vi "Begin.vi"() -> (0 "error out":errorcluster, 1 "error out 2":errorcluster)   [LabVIEW 2013]
doc: "Called before other user functions, this VI is expected to open initial I/O refnums, load in file data, and do all program initialization. Notice that the <B>error out</B> terminal is simply used for data flow. Wiring it to other structures or subVIs ensures that this VI runs first."
uses:
  <vilib>/Rock Robotics/WPI/DriverStation/WPI_DriverStationRobotMode2.ctl
  <vilib>/Rock Robotics/SystemInterfaces/DIO/FPGA_DIOPWMChannel.ctl
  <vilib>/Rock Robotics/WPI/SafetyOutput/WPI_SafetyOutputConfigMenu.ctl
  <vilib>/Rock Robotics/WPI/Joystick/WPI_JoystickDeviceEnum.ctl
  <vilib>/Rock Robotics/SystemInterfaces/Typedef/FPGA_TypedefDigitalModule.ctl
  <vilib>/Rock Robotics/WPI/Solenoid/WPI_SolenoidChannel.ctl
  <vilib>/Rock Robotics/SystemInterfaces/DIO/FPGA_DIORelayChannel.ctl
  <vilib>/Rock Robotics/SystemInterfaces/DIO/FPGA_DIOChannel.ctl
  <vilib>/Rock Robotics/SystemInterfaces/AI/FPGA_AIChannel.ctl
  <vilib>/Rock Robotics/SystemInterfaces/Typedef/FPGA_TypedefAnalogModule.ctl
  <vilib>/Rock Robotics/WPI/Relay/WPI_RelayValue.ctl
  <vilib>/Rock Robotics/WPI/Relay/WPI_RelayDirection.ctl
  <vilib>/Rock Robotics/SystemInterfaces/Typedef/FPGA_TypedefSolenoidModule.ctl
  <vilib>/Rock Robotics/WPI/Solenoid/WPI_SolenoidValue.ctl
  Robot Global Data.vi
  <vilib>/Rock Robotics/WPI/RobotDrive/WPI_RobotDriveOpen2MotorWithTalon.vi
  <vilib>/Rock Robotics/WPI/MotorControl/WPI_MotorControlOpen Jaguar.vi
  <vilib>/Rock Robotics/WPI/Solenoid/WPI_SolenoidOpenDouble.vi
  <vilib>/Rock Robotics/WPI/MotorControl/WPI_MotorControlOpen Talon.vi
  <vilib>/Rock Robotics/WPI/Solenoid/WPI_SolenoidOpenSingle.vi
  <vilib>/Rock Robotics/WPI/Solenoid/WPI_SolenoidGetEnum.vi
  <vilib>/Rock Robotics/WPI/Solenoid/WPI_SolenoidSetEnum.vi
  <vilib>/Rock Robotics/WPI/Compressor/WPI_CompressorGetSetRefNum.vi
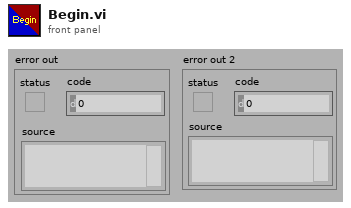
[diagram p1: front panel]
types:
  T1 = typedef "WPI_SolenoidValue.ctl" = enum16{"Off", "On", "Forward", "Reverse"}
  T2 = typedef "WPI_SolenoidChannel.ctl" = enum8{"Solenoid 1", "Solenoid 2", "Solenoid 3", "Solenoid 4", "Solenoid 5", "Solenoid 6", "Solenoid 7", "Solenoid 8", "Invalid"}
  T3 = typedef "FPGA_TypedefSolenoidModule.ctl" = enum16{"Solenoid Module 1", "Solenoid Module 2"}
  T4 = typedef "WPI_RelayDirection.ctl" = enum16{"Both directions", "Forward only", "Reverse only"}
  T5 = typedef "FPGA_DIORelayChannel.ctl" = enum8{"Relay 1", "Relay 2", "Relay 3", "Relay 4", "Relay 5", "Relay 6", "Relay 7", "Relay 8", "Invalid"}
  T6 = typedef "FPGA_TypedefDigitalModule.ctl" = enum16{"Digital Module 1", "Digital Module 2"}
  T7 = typedef "WPI_RelayValue.ctl" = enum16{"Off", "On", "Forward", "Reverse"}
  T8 = typedef "FPGA_DIOChannel.ctl" = enum8{"DIO 1", "DIO 2", "DIO 3", "DIO 4", "DIO 5", "DIO 6", "DIO 7", "DIO 8", "DIO 9", "DIO 10", "DIO 11", "DIO 12", "DIO 13", "DIO 14", "Invalid"}
  T9 = typedef "FPGA_AIChannel.ctl" = enum8{"AI 1", "AI 2", "AI 3", "AI 4", "AI 5", "AI 6", "AI 7", "AI 8", "Invalid"}
  T10 = typedef "FPGA_TypedefAnalogModule.ctl" = enum16{"Analog Module 1", "Analog Module 2"}
  T11 = typedef "FPGA_DIOPWMChannel.ctl" = enum8{"PWM 1", "PWM 2", "PWM 3", "PWM 4", "PWM 5", "PWM 6", "PWM 7", "PWM 8", "PWM 9", "PWM 10", "Invalid"}
  T12 = typedef "WPI_JoystickDeviceEnum.ctl" = enum16{"USB 1", "USB 2", "USB 3", "USB 4", "Kinect 1", "Kinect 2"}
  T13 = typedef "WPI_SafetyOutputConfigMenu.ctl" = enum16{"Enable", "Disable"}
  T14 = typedef "WPI_DriverStationRobotMode2.ctl" = enum16{"Autonomous Disabled", "Autonomous Enabled", "Teleop Disabled", "Teleop Enabled", "Timeout", "Finish", "Test Disabled", "Test Enabled"}
  T15 = typedef "WPI_MotorControlDeviceRef.ctl" = cluster{"DeviceStatus":errorcluster, "Type":enum16{"PWM", "CAN"}, "PWM":cluster{"Digital Module":T6, "PWM Channel":T11, "DeadBand":T16}, "CAN":cluster{"Device Number":u8, "Control Mode":T17, "Semaphore":T18, "Max Vout":dbl}, "Invert":bool, "TransformRef":T19, "InvTransformRef":T19}
  T16 = typedef "WPI_PWMDeadband.ctl" = cluster{"Name":string, "maxPositivePwm":i32, "minPositivePwm":i32, "centerPwm":i32, "maxNegativePwm":i32, "minNegativePwm":i32, "angularRange":u16}
  T17 = typedef "WPI_CANJaguar_ControlMode.ctl" = enum8{"Percent VBus", "Current", "Speed", "Position", "Voltage"}
  T18 = typedef "Semaphore RefNum" = refnum<k1>
  T19 = typedef "WPI_PWMTransform_ConPane.ctl" = refnum<vi>
  T20 = typedef "WPI_JoystickDevRef.ctl" = cluster{"Device":T12}
  T21 = typedef "WPI_DigitalInputDevRef.ctl" = cluster{"DevStatus":errorcluster, "DIO Channel":T8, "Digital Module":T6}
  T22 = typedef "WPI_RobotDriveDevRef.ctl" = cluster{"DevStatus":errorcluster, "Motors[]":T15[], "Square Inputs":bool, "Max Output":dbl, "Isochronous":bool}
  T23 = typedef "WPI_SolenoidDevRef.ctl" = cluster{"DevStatus":errorcluster, "Solenoid Module":T3, "Forward Solenoid Channel":T2, "Reverse Solenoid Channel":T2}
  T24 = typedef "WPI_RelayDevRef.ctl" = cluster{"DevStatus":errorcluster, "Relay Channel":T5, "Digital Module":T6, "Relay Direction":T4}
  T25 = typedef "WPI_CompressorDevRef.ctl" = cluster{"DevStatus":errorcluster, "DigitalInputDevRef":T21, "RelayDevRef":T24}
  T26 = typedef "WPI_AnalogChannelDevRef.ctl" = cluster{"DevStatus":errorcluster, "Analog Module":T10, "Analog Channel":T9}
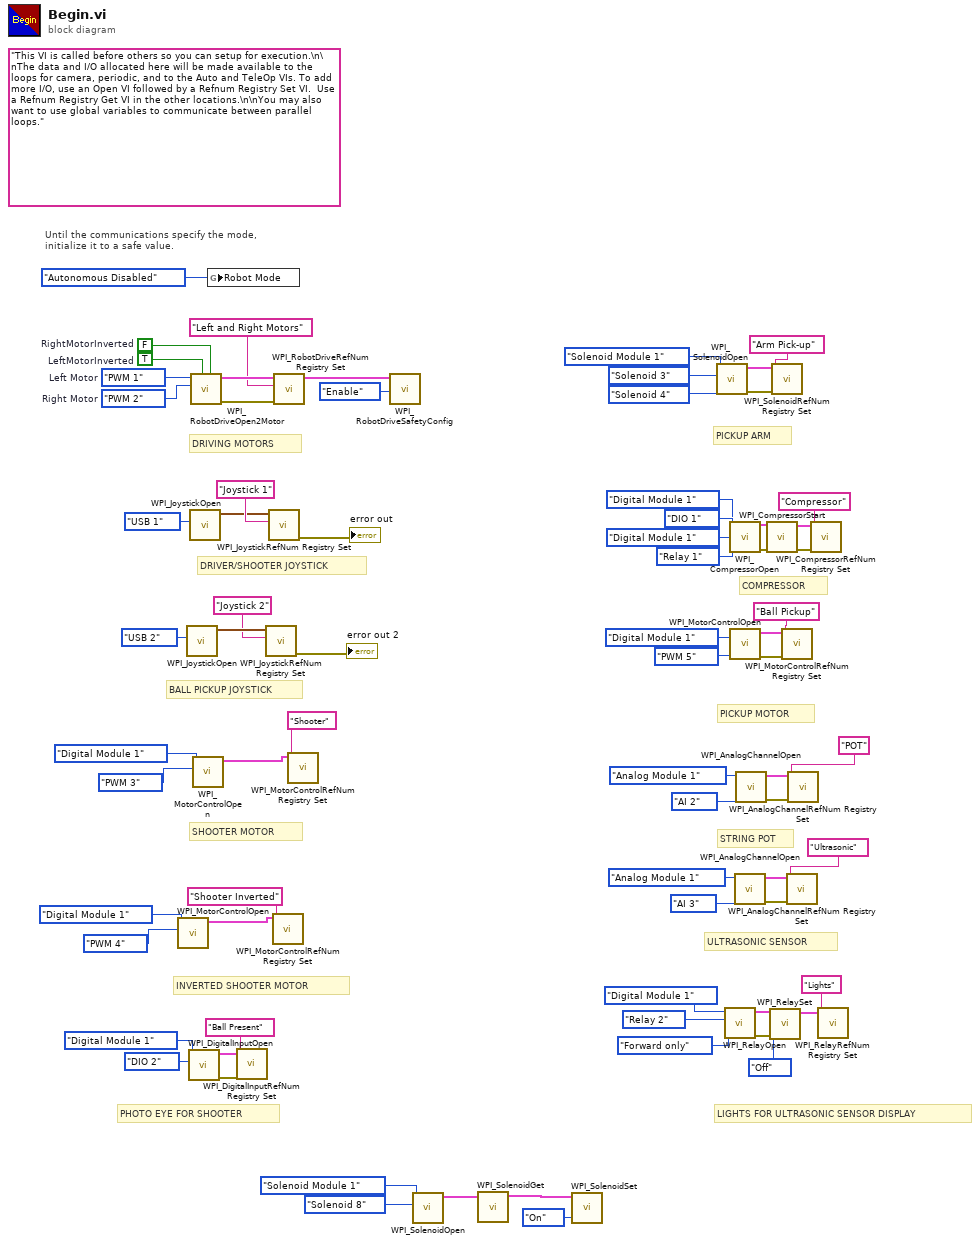
[diagram p0: block diagram]
diagram:
  w67 = FPGA_DIOPWMChannel."PWM 2"  # Right Motor
  w68 = FPGA_DIOPWMChannel."PWM 1"  # Left Motor
  w72 = TRUE  # LeftMotorInverted
  w73 = FALSE  # RightMotorInverted
  (unwired) "This VI is called before others so you can setup for execution.\n\nThe data and I/O allocated here will be made available to the loops for camera, periodic, and to the Auto and TeleOp VIs. To add more I/O, use an Open VI followed by a Refnum Registry Set VI.  Use a Refnum Registry Get VI in the other locations.\n\nYou may also want to use global variables to communicate between parallel loops."
  # "LIGHTS FOR ULTRASONIC SENSOR DISPLAY"
  # "PHOTO EYE FOR SHOOTER"
  # "ULTRASONIC SENSOR"
  # "STRING POT"
  # "PICKUP MOTOR"
  # "COMPRESSOR"
  # "PICKUP ARM"
  # "INVERTED SHOOTER MOTOR"
  # "SHOOTER MOTOR"
  # "BALL PICKUP JOYSTICK"
  # "DRIVER/SHOOTER JOYSTICK"
  # "DRIVING MOTORS"
  # "Until the communications specify the mode,\ninitialize it to a safe value."
  n1 = call-poly <vilib>:"WPI_MotorControlOpen.vi"("PWM Channel"=FPGA_DIOPWMChannel."PWM 4", "Digital Module (Module 1)"=FPGA_TypedefDigitalModule."Digital Module 1") -> ("MotorControlDeviceRef"=w51:T15)  [unwired: 8 in, 1 out]
  n2 = call <vilib>:"WPI_JoystickOpen.vi"("JoystickDevice"=WPI_JoystickDeviceEnum."USB 2") -> ("JoystickDevRef"=w58:T20)  [unwired: 10 in]
  n3 = call <vilib>:"WPI_DigitalInputOpen.vi"("DIO Channel"=FPGA_DIOChannel."DIO 2", "Digital Module (Module 1)"=FPGA_TypedefDigitalModule."Digital Module 1") -> ("error out"=w16:errorcluster, "DigitalInputDevRef"=w15:T21)  [unwired: 8 in]
  n4 = call <vilib>:"WPI_JoystickOpen.vi"("JoystickDevice"=WPI_JoystickDeviceEnum."USB 1") -> ("JoystickDevRef"=w63:T20)  [unwired: 10 in]
  n5 = call-poly <vilib>:"WPI_RobotDriveOpen2Motor.vi"("Right Motor Inverted"=w73, "Left Motor Inverted"=w72, "Right Motor"=w67, "Left Motor"=w68) -> ("error out"=w69:errorcluster, "RobotDriveDevRef"=w71:T22)  [unwired: 1 in, 5 out]
  n6 = call-poly <vilib>:"WPI_MotorControlOpen.vi"("PWM Channel"=FPGA_DIOPWMChannel."PWM 3", "Digital Module (Module 1)"=FPGA_TypedefDigitalModule."Digital Module 1") -> ("MotorControlDeviceRef"=w56:T15)  [unwired: 8 in, 1 out]
  n7 = global write "Robot Global Data.vi" "Robot Mode"(WPI_DriverStationRobotMode2."Autonomous Disabled" ("Robot Mode")) -> ()
  n8 = call <vilib>:"WPI_DigitalInputRefNum Registry Set.vi"("error in (no error)"=w16, "refnum name"="Ball Present", "DigitalInputDevRef"=w15) -> ()  [unwired: 7 in, 2 out]
  n9 = call <vilib>:"WPI_JoystickRefNum Registry Set.vi"("refnum name"="Joystick 2", "JoystickDevRef"=w58) -> ("error out"=→"error out 2":errorcluster)  [unwired: 8 in, 1 out]
  n10 = call <vilib>:"WPI_JoystickRefNum Registry Set.vi"("refnum name"="Joystick 1", "JoystickDevRef"=w63) -> ("error out"=→"error out":errorcluster)  [unwired: 8 in, 1 out]
  n11 = call <vilib>:"WPI_MotorControlRefNum Registry Set.vi"("refnum name"="Shooter Inverted", "MotorControlDevRef"=w51) -> ()  [unwired: 8 in, 2 out]
  n12 = call <vilib>:"WPI_RobotDriveRefNum Registry Set.vi"("error in (no error)"=w69, "refnum name"="Left and Right Motors", "RobotDriveDevRef"=w71) -> ("RobotDriveDevRef"=w66:T22)  [unwired: 8 out]
  n13 = call <vilib>:"WPI_MotorControlRefNum Registry Set.vi"("refnum name"="Shooter", "MotorControlDevRef"=w56) -> ()  [unwired: 8 in, 2 out]
  n14 = call <vilib>:"WPI_RobotDriveSafetyConfig.vi"("mode"=WPI_SafetyOutputConfigMenu."Enable", "RobotDriveDevRef"=w66) -> ()  [unwired: 8 in, 2 out]
  n15 = call-poly <vilib>:"WPI_SolenoidOpen.vi"("Solenoid Channel"=WPI_SolenoidChannel."Solenoid 8" ("Forward Solenoid Channel"), "Solenoid Module (Module 1)"=FPGA_TypedefSolenoidModule."Solenoid Module 1") -> ("SolenoidDevRef"=w3:T23)  [unwired: 8 in, 1 out]
  n16 = call-poly <vilib>:"WPI_SolenoidGet.vi"("SolenoidDevRef"=w3) -> ("SolenoidDevRef"=w2:T23)  [unwired: 8 in, 2 out]
  n17 = call-poly <vilib>:"WPI_SolenoidSet.vi"("Value"=WPI_SolenoidValue."On", "SolenoidDevRef"=w2) -> ()  [unwired: 8 in, 2 out]
  n18 = call-poly <vilib>:"WPI_SolenoidOpen.vi"("Reverse Solenoid Channel"=WPI_SolenoidChannel."Solenoid 4", "Forward Solenoid Channel"=WPI_SolenoidChannel."Solenoid 3", "Solenoid Module (Module 1)"=FPGA_TypedefSolenoidModule."Solenoid Module 1") -> ("error out"=w45:errorcluster, "SolenoidDevRef"=w44:T23)  [unwired: 7 in]
  n19 = call <vilib>:"WPI_RelayOpen.vi"("Relay Direction"=WPI_RelayDirection."Forward only", "Relay Channel"=FPGA_DIORelayChannel."Relay 2", "Digital Module (Module 1)"=FPGA_TypedefDigitalModule."Digital Module 1") -> ("error out"=w13:errorcluster, "RelayDevRef"=w12:T24)  [unwired: 7 in]
  n20 = call <vilib>:"WPI_CompressorOpen.vi"("Pressure Switch Digital Module (Module 1)"=FPGA_TypedefDigitalModule."Digital Module 1", "Pressure Switch DIO Channel"=FPGA_DIOChannel."DIO 1", "Relay Digital Module (Module 1)"=FPGA_TypedefDigitalModule."Digital Module 1", "Relay Channel"=FPGA_DIORelayChannel."Relay 1") -> ("CompressorDevRef"=w39:T25, "error out"=w40:errorcluster)  [unwired: 10 in]
  n21 = call-poly <vilib>:"WPI_MotorControlOpen.vi"("PWM Channel"=FPGA_DIOPWMChannel."PWM 5", "Digital Module (Module 1)"=FPGA_TypedefDigitalModule."Digital Module 1") -> ("error out"=w33:errorcluster, "MotorControlDeviceRef"=w32:T15)  [unwired: 8 in]
  n22 = call <vilib>:"WPI_AnalogChannelOpen.vi"("Analog Channel"=FPGA_AIChannel."AI 3", "Analog Module (Module 1)"=FPGA_TypedefAnalogModule."Analog Module 1") -> ("error out"=w21:errorcluster, "AIDeviceRef"=w22:T26)  [unwired: 8 in]
  n23 = call <vilib>:"WPI_AnalogChannelOpen.vi"("Analog Channel"=FPGA_AIChannel."AI 2", "Analog Module (Module 1)"=FPGA_TypedefAnalogModule."Analog Module 1") -> ("error out"=w26:errorcluster, "AIDeviceRef"=w25:T26)  [unwired: 8 in]
  n24 = call <vilib>:"WPI_CompressorStart.vi"("error in (no error)"=w40, "CompressorDevRef"=w39) -> ("error out"=w38:errorcluster, "CompressorDevRef"=w37:T25)  [unwired: 8 in]
  n25 = call <vilib>:"WPI_RelaySet.vi"("error in (no error)"=w13, "RelayValue"=WPI_RelayValue."Off", "RelayDevRef"=w12) -> ("RelayDevRef"=w10:T24)  [unwired: 7 in, 1 out]
  n26 = call <vilib>:"WPI_SolenoidRefNum Registry Set.vi"("error in (no error)"=w45, "refnum name"="Arm Pick-up", "SolenoidDevRef"=w44) -> ()  [unwired: 7 in, 2 out]
  n27 = call <vilib>:"WPI_MotorControlRefNum Registry Set.vi"("error in (no error)"=w33, "refnum name"="Ball Pickup", "MotorControlDevRef"=w32) -> ()  [unwired: 7 in, 2 out]
  n28 = call <vilib>:"WPI_AnalogChannelRefNum Registry Set.vi"("error in (no error)"=w21, "refnum name"="Ultrasonic", "AIDeviceRef"=w22) -> ()  [unwired: 7 in, 2 out]
  n29 = call <vilib>:"WPI_AnalogChannelRefNum Registry Set.vi"("error in (no error)"=w26, "refnum name"="POT", "AIDeviceRef"=w25) -> ()  [unwired: 7 in, 2 out]
  n30 = call <vilib>:"WPI_CompressorRefNum Registry Set.vi"("error in (no error)"=w38, "refnum name"="Compressor", "CompressorDevRef"=w37) -> ()  [unwired: 7 in, 2 out]
  n31 = call <vilib>:"WPI_RelayRefNum Registry Set.vi"("refnum name"="Lights", "RelayDevRef"=w10) -> ()  [unwired: 8 in, 2 out]
